vi "Teardown.vi"(8 "Error In":errorcluster, 11 "Renderer":refnum<class "Renderer.lvclass">) -> (0 "Error Out":errorcluster, 3 "Output":string)   [LabVIEW 2018, in "Tests.lvlib" / "Render.lvlib"]
uses:
  Render.lvlib
  src/Toolkit/Low-Level/Renderer/Renderer.lvclass
  src/Toolkit/Low-Level/Writers/String/String.lvclass
  src/Toolkit/Low-Level/Writers/String/String.lvclass/String.ctl
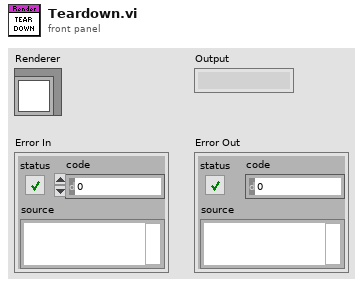
[diagram p1: front panel]
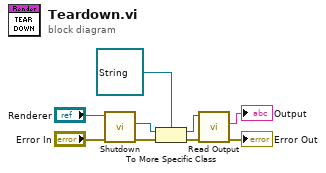
[diagram p0: block diagram]
diagram:
  n1 = call-dynamic "Shutdown.vi"("Error In"="Error In", "Renderer In"="Renderer") -> ("Error Out"=w2:errorcluster, "Writer"=w1:refnum<class "Writer.lvclass">)  [unwired: 5 in, 3 out]
  n2 = To More Specific Class(target class=refnum<class "String.lvclass"> refnum ("Toolkit.lvlib:Writers.lvlib:String.lvclass"), reference=w1, error in=w2) -> (specific class reference=w3:refnum<class "String.lvclass">, error out=w7:errorcluster)
  n3 = call "Read Output.vi"("Error In"=w7, "String In"=w3) -> ("Error Out"=→"Error Out":errorcluster, "Output"=→"Output":string)  [unwired: 7 in, 1 out]
